vi "SavPath.vi"() -> ()   [LabVIEW 2011]
panel:
  in  "SavePath":path
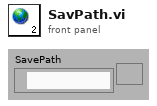
[diagram p1: front panel]
diagram:
